vi "Is Valid Reference.vi"(11 "Reference":refnum<vi>) -> (3 "Reference Is Valid":bool)   [LabVIEW 2013]
uses:
  Command Processor/Command/Command Status.ctl
  Command Processor/Command/State Status.ctl
  Command Processor/Command/Command.lvclass
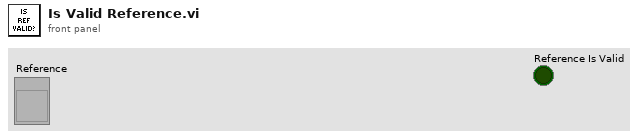
[diagram p1: front panel]
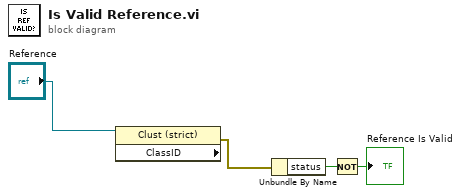
[diagram p0: block diagram]
diagram:
  n1 = property class="Clust (strict)" props=["ClassID"](reference="Reference") -> (error out=w3:errorcluster)  [unwired: 1 in, 2 out]
  n2 = Unbundle By Name(w3) -> ("status"=w2:bool)
  n3 = Not(x=w2) -> (.not. x?=→"Reference Is Valid":bool)
